vi "Read Props.vi"(8 "error in (no error)":errorcluster, 11 "SimpleGraphEditorPanel in":refnum<class "SimpleGraphEditorPanel.lvclass">) -> (0 "error out":errorcluster, 2 "Props":T1, 3 "SimpleGraphEditorPanel out":refnum<class "SimpleGraphEditorPanel.lvclass">)   [LabVIEW 2020, in "VolatusGUIControls.lvlib" / "SimpleGraphEditorPanel.lvclass"]
uses:
  SimpleGraphEditorPanel.lvclass
  SimpleGraphEditorPanel.lvclass/SimpleGraphEditorPanel.ctl
  VolatusGUIControls.lvlib
  50fbb230-99c1-41c9-94d9-f9da72bf3217.vi
  JSON Props.ctl
  VolatusGUIEditorCore/Position Props.ctl
  VolatusGUIEditorCore/VolatusGUIEditorCore.lvlib
  Props.ctl
  VolatusGUIEditorCore/Label Props.ctl
  VolatusGUIEditorCore/Plot Legend Props.ctl
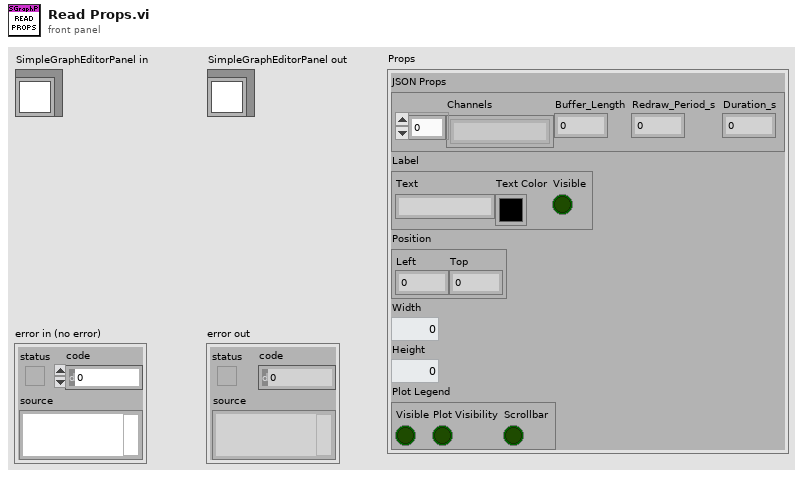
[diagram p1: front panel]
types:
  T1 = typedef "VolatusGUIControls.lvlib/SimpleGraphEditorPanel.lvclass/Props.ctl" = cluster{"JSON Props":T2, "Label":T3, "Position":T4, "Width":u16, "Height":u16, "Plot Legend":T5}
  T2 = typedef "VolatusGUIControls.lvlib/SimpleGraphEditorPanel.lvclass/JSON Props.ctl" = cluster{"Channels":string[], "Buffer_Length":i32, "Redraw_Period_s":dbl, "Duration_s":i32}
  T3 = typedef "VolatusGUIEditorCore.lvlib/Label Props.ctl" = cluster{"Text":string, "Text Color":u32, "Visible":bool}
  T4 = typedef "VolatusGUIEditorCore.lvlib/Position Props.ctl" = cluster{"Left":i32, "Top":i32}
  T5 = typedef "VolatusGUIEditorCore.lvlib/Plot Legend Props.ctl" = cluster{"Visible":bool, "Plot Visibility":bool, "Scrollbar":bool}
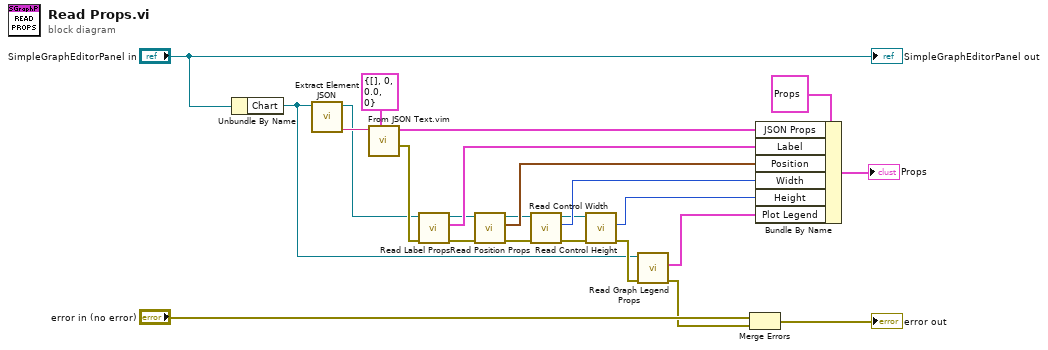
[diagram p0: block diagram]
diagram:
  n1 = Unbundle By Name("SimpleGraphEditorPanel in") -> ("Chart"=w3:refnum<vi>)
  n2 = call "Extract Element JSON.vi"("Ctl Refnum in"=w3) -> ("JSON"=w20:string, "Ctl Refnum"=w16:refnum<vi>)  [unwired: 7 in, 2 out]
  n3 = call "From JSON Text.vim"("Data Type and Default Value"=T2 {"Channels"=[], "Buffer_Length"=0, "Redraw_Period_s"=0.0, "Duration_s"=0} ("JSON Props"), "JSON"=w20) -> ("error out"=w23:errorcluster, "Data out"=w4:T2)  [unwired: 8 in]
  n4 = call "Read Label Props.vi"("error in (no error)"=w23, "Ctl Refnum in"=w16) -> ("error out"=w13:errorcluster, "Label Props"=w15:T3, "Ctl Refnum"=w14:refnum<vi>)  [unwired: 7 in]
  n5 = call "Read Position Props.vi"("error in (no error)"=w13, "Ctl Refnum in"=w14) -> ("error out"=w11:errorcluster, "Position Props"=w12:T4, "Ctl Refnum"=w10:refnum<vi>)  [unwired: 7 in]
  n6 = call "Read Control Width.vi"("error in"=w11, "Control in"=w10) -> ("error out"=w8:errorcluster, "Width"=w9:u32, "Control"=w7:refnum<vi>)  [unwired: 7 in]
  n7 = call "Read Control Height.vi"("error in"=w8, "Control in"=w7) -> ("error out"=w24:errorcluster, "Height"=w6:u32)  [unwired: 7 in, 1 out]
  n8 = call "Read Graph Legend Props.vi"("error in (no error)"=w24, "Graph in"=w3) -> ("error out"=w2:errorcluster, "Plot Legend Props"=w1:T5)  [unwired: 7 in, 1 out]
  n9 = Merge Errors("error in (no error)", w2) -> (→"error out":errorcluster)
  n10 = Bundle By Name(cluster=T1 {"JSON Props"={"Channels"=[], "Buffer_Length"=0, "Redraw_Period_s"=0.0, "Duration_s"=0}, "Label"={"Text"="", "Text Color"=0, "Visible"=FALSE}, "Position"={"Left"=0, "Top"=0}, "Width"=0, "Height"=0, "Plot Legend"={"Visible"=FALSE, "Plot Visibility"=FALSE, "Scrollbar"=FALSE}} ("Props"), "JSON Props"=w4, "Label"=w15, "Position"=w12, "Width"=w9, "Height"=w6, "Plot Legend"=w1) -> (→"Props":T1)
  "SimpleGraphEditorPanel out" <- "SimpleGraphEditorPanel in"
